vi "Is Site in Map.vi"(8 "error in":errorcluster, 10 "site":i32, 11 "connection map in":refnum<class "Connection Map.lvclass">) -> (0 "error out":errorcluster, 2 "site in map":bool, 3 "connection map out":refnum<class "Connection Map.lvclass">)   [LabVIEW 2020, in "MeasurementLink Session Management.lvlib" / "Connection Map.lvclass"]
uses:
  Connection Map.lvclass
  Connection Map.lvclass/Connection Map.ctl
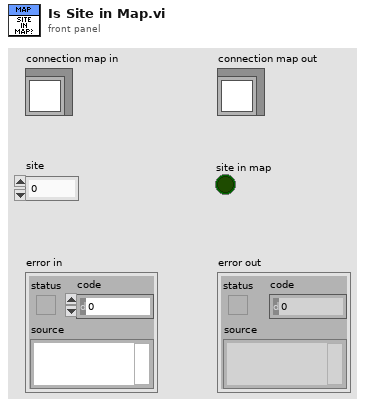
[diagram p1: front panel]
types:
  T1 = typedef "MeasurementLink Session Management.lvlib/Session Reservation.lvclass/Connection with Session.ctl" = cluster{"connection":T2, "session":variant}
  T2 = typedef "MeasurementLink Session Management.lvlib/Session Reservation.lvclass/Connection.ctl" = cluster{"pin or relay name":string, "site":i32, "instrument type id":string, "channel":string}
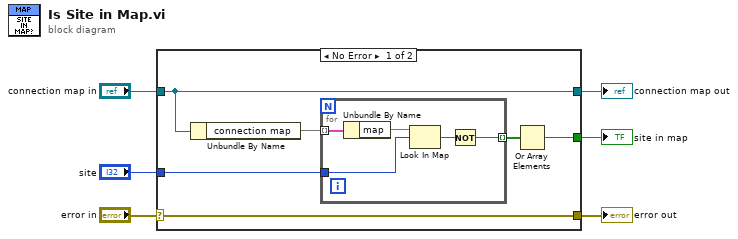
[diagram p0: block diagram]
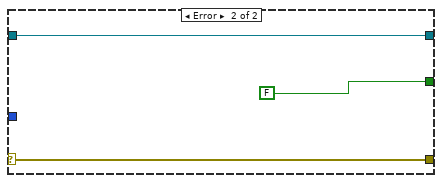
[diagram p2: hidden frame]
diagram:
  n1 = case shown="No Error" "error in" {
    selector: "error in" -> [w12 w20]
    tunnel: [w12 w20] -> w5
    tunnel: [w11 w19] -> w3
    tunnel: "connection map in" -> [w11 w19]
    tunnel: "site" -> [w9 _]
    tunnel: [w7 FALSE ("key not found?")] -> w1
    frame No Error {
      n2 = Unbundle By Name(w11) -> ("connection map"=w10:map{string, map{i32, map{string, T1}}})
      n3 = for {
        tunnel: w10 -> [w17] mode=indexing
        tunnel: w9 -> [w15]
        tunnel: [w13] -> w8 mode=indexing
        n4 = Unbundle By Name(w17) -> ("map"=w16:map{i32, map{string, T1}})
        n5 = Look In Map(map=w16, key=w15) -> (key not found?=w14:bool)  [unwired: 1 in, 1 out]
        n6 = Not(x=w14) -> (.not. x?=w13:bool)
      }
      n7 = Or Array Elements(Boolean array=w8) -> (logical OR=w7:bool)
    }
    frame Error {
    }
  }
  "error out" <- w5
  "connection map out" <- w3
  "site in map" <- w1
